vi "CalcAngleCircle.vi"(0 "Original Image":T1(plugin-control), 1 "Filtered Image":T1(plugin-control), 2 "X Coordinate":i32=322, 3 "Y Coordinate":i32=238, 4 "Vertical radius":i32) -> (5 "Angle in degrees":dbl)   [LabVIEW 2009, in "ImageAnalysis.lvlib"]
uses:
  ImageAnalysis.lvlib
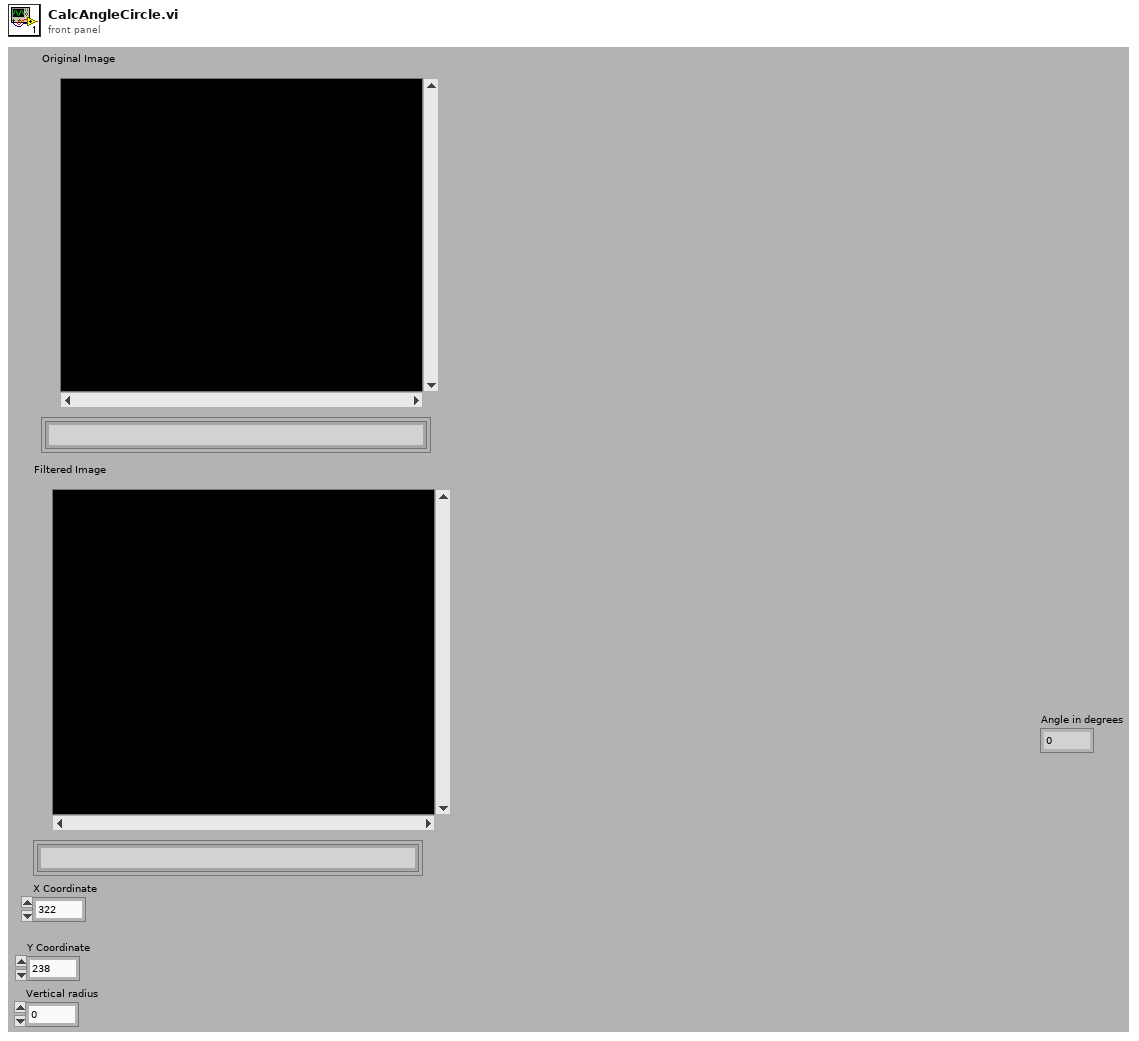
[diagram p1: front panel]
types:
  T1 = typedef "IMAQ Image.ctl" = refnum<image>
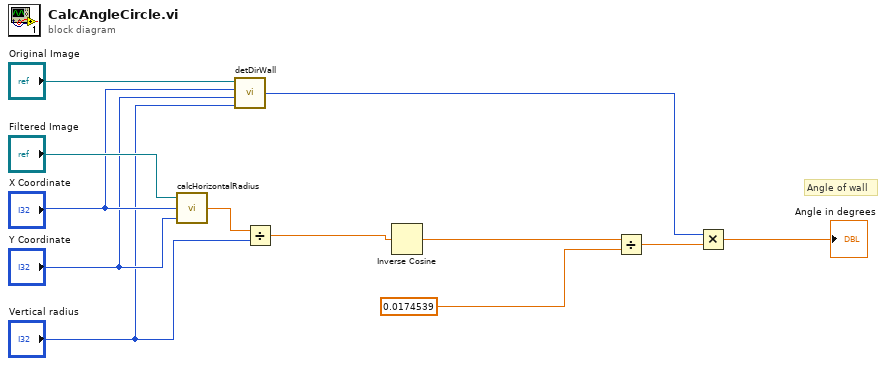
[diagram p0: block diagram]
diagram:
  # "Angle of wall"
  n1 = call "calcHorizontalRadius.vi"("Y Coordinate"="Y Coordinate", "X Coordinate"="X Coordinate", "Source Image"="Filtered Image") -> ("mean radius"=w6:dbl)
  n2 = call "detDirWall.vi"("Radius"="Vertical radius", "Y-cord"="Y Coordinate", "X-cord"="X Coordinate", "Source Image"="Original Image") -> ("Angle dir"=w9:i32)
  n3 = Divide(x=w6, y="Vertical radius") -> (x/y=w12:dbl)
  n4 = Inverse Cosine(1:w12) -> (0:w11:dbl)
  n5 = Divide(x=w11, y=0.0174539) -> (x/y=w8:dbl)
  n6 = Multiply(x=w9, y=w8) -> (x*y=→"Angle in degrees":dbl)
